vi "PIDF Internal.vi"(4 "PID State":T1, 5 "invert? (F)":bool, 6 "PIDF gains":cluster{"Kp":dbl, "Ki":dbl, "Kd":dbl, "Kf":dbl} {"Kf" format="%.3f"; "Kd" format="%.3f"; "Ki" format="%.3f"; "Kp" format="%.3f"}, 7 "output range":cluster{"output high":dbl, "output low":dbl}={"output high"=1.0, "output low"=-1.0} {"output low" format="%.2f"; "output high" format="%.2f"}, 8 "dt (s)":dbl=0.01, 9 "i Zone":dbl=inf format="%.2f", 10 "process variable":dbl format="%.2f", 11 "setpoint":dbl format="%.2f") -> (0 "In i Zone?":bool, 1 "In Range?":bool, 2 "output":dbl format="%.2f", 3 "PID State":T1)   [LabVIEW 2019]
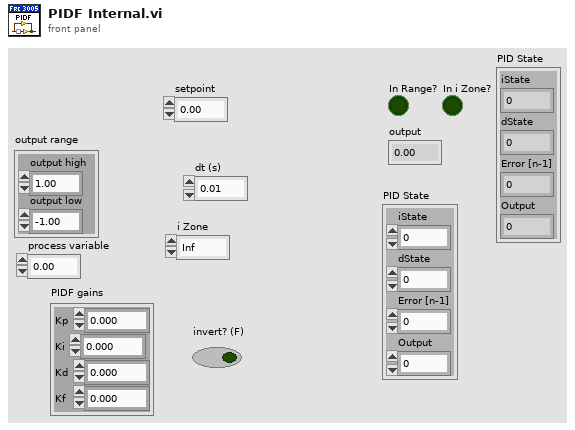
[diagram p1: front panel]
types:
  T1 = cluster{"iState":dbl, "dState":dbl, "Error [n-1]":dbl, "Output":dbl}
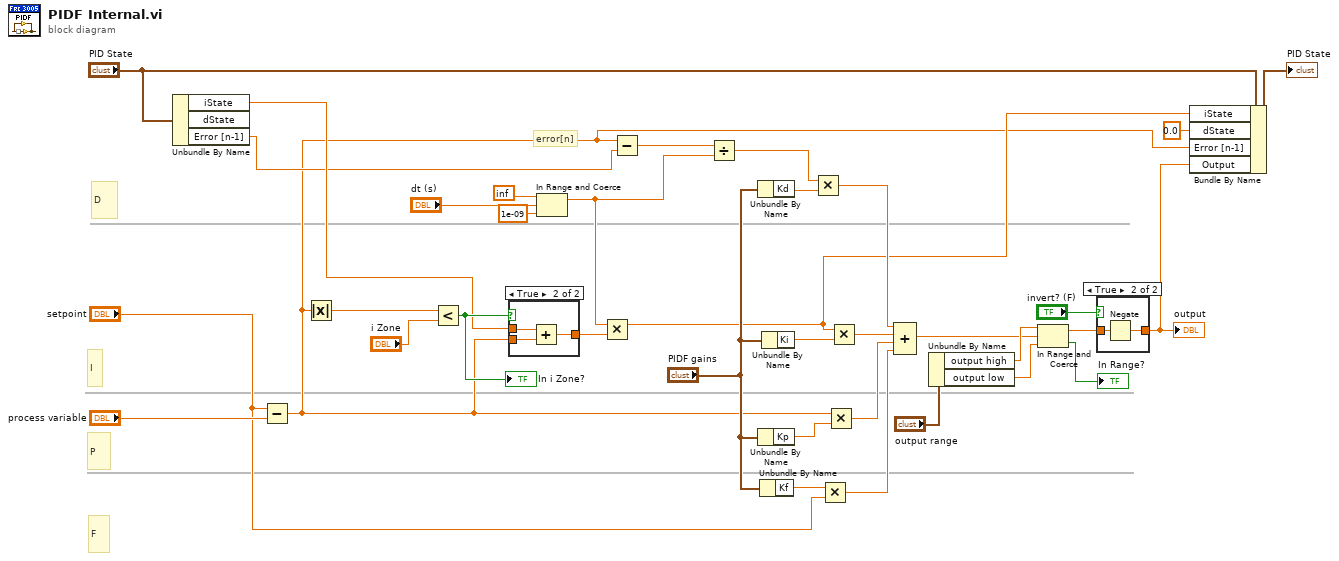
[diagram p0: block diagram]
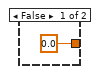
[diagram p3: hidden frame]
diagram:
  # "F"
  # "D"
  # "I"
  # "P"
  # "error[n]"
  n1 = Unbundle By Name("PID State") -> ("iState"=w5:dbl, "Error [n-1]"=w4:dbl)  [unwired: 1 out]
  n2 = Subtract(x="setpoint", y="process variable") -> (x-y=w2:dbl)
  n3 = Absolute Value(x=w2) -> (abs(x)=w34:dbl)
  n4 = Less?(x=w34, y="i Zone") -> (x < y?=w32:bool)
  "In i Zone?" <- w32
  n5 = case shown="True" w32 {
    tunnel: w2 -> [_ w40]
    tunnel: [0.0 ("f") w39] -> w12
    tunnel: w5 -> [_ w38]
    frame False {
    }
    frame True {
      n6 = Add(x=w38, y=w40) -> (x+y=w39:dbl)
    }
  }
  n7 = In Range and Coerce(upper limit=inf, x="dt (s)", lower limit=1e-09) -> (coerced(x)=w8:dbl)  [unwired: 1 out]
  n8 = Multiply(x=w8, y=w12) -> (x*y=w13:dbl)
  n9 = Subtract(x=w2, y=w4) -> (x-y=w15:dbl)
  n10 = Divide(x=w15, y=w8) -> (x/y=w14:dbl)
  n11 = Unbundle By Name("PIDF gains") -> ("Kd"=w23:dbl)
  n12 = Unbundle By Name("PIDF gains") -> ("Kp"=w35:dbl)
  n13 = Unbundle By Name("PIDF gains") -> ("Kf"=w25:dbl)
  n14 = Unbundle By Name("PIDF gains") -> ("Ki"=w21:dbl)
  n15 = Multiply(x=w14, y=w23) -> (x*y=w22:dbl)
  n16 = Multiply(x=w25, y="setpoint") -> (x*y=w24:dbl)
  n17 = Multiply(x=w2, y=w35) -> (x*y=w31:dbl)
  n18 = Multiply(x=w13, y=w21) -> (x*y=w20:dbl)
  n19 = Compound Arithmetic op=ADD(w22, w20, w31, w24) -> (w27:dbl)
  n20 = Unbundle By Name("output range") -> ("output high"=w29:dbl, "output low"=w28:dbl)
  n21 = In Range and Coerce(upper limit=w29, x=w27, lower limit=w28) -> (coerced(x)=w18:dbl, In Range?=→"In Range?":bool)
  n22 = case shown="True" "invert? (F)" {
    tunnel: w18 -> [w41 w43]
    tunnel: [w41 w42] -> w3
    frame False {
    }
    frame True {
      n23 = Negate(x=w43) -> (-x=w42:dbl)
    }
  }
  "output" <- w3
  n24 = Bundle By Name(cluster="PID State", "iState"=w13, "dState"=0.0, "Error [n-1]"=w2, "Output"=w3) -> (→"PID State":T1)
